vi "AVQ8347 Wavelike Data_backslash_n.vi"(0 "VISA Session":refnum<visa-resource-name>, 1 "Axis Select":T1(ring), 5 "Error In":errorcluster) -> (14 "Copy VISA Session":refnum<visa-resource-name>, 15 "Return All Data":string, 16 "Wavelike Data":dbl[](array[numeric]) format="%.12f", 17 "Return Data Bytes":u16, 19 "Error Out":errorcluster)   [LabVIEW 2020]
doc: "This function returns the wavelike data value\n\n(NEC-PC Mode Data is Return All Data Only)"
panel:
  out "CntWk":u16
  out "String Work":string
  # "Wavelike Data"
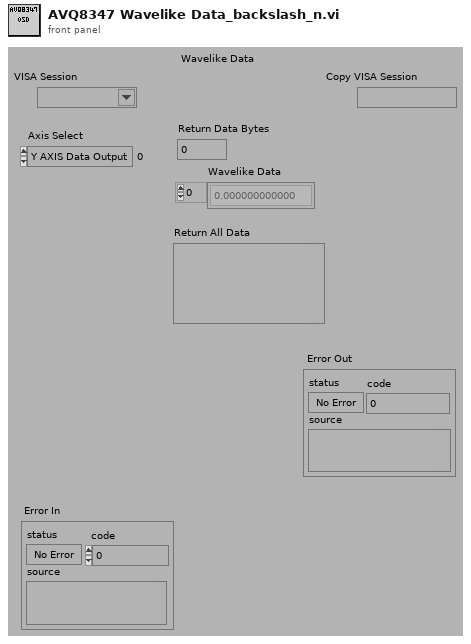
[diagram p1: front panel]
types:
  T1 = enum16{"Y AXIS Data Output", "X AXIS Data Output"}
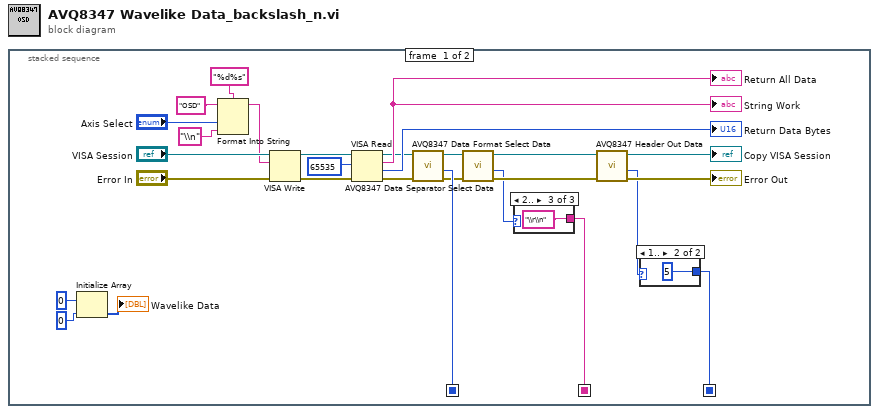
[diagram p0: block diagram]
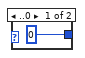
[diagram p2: hidden frame]
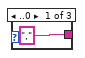
[diagram p3: hidden frame]
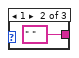
[diagram p4: hidden frame]
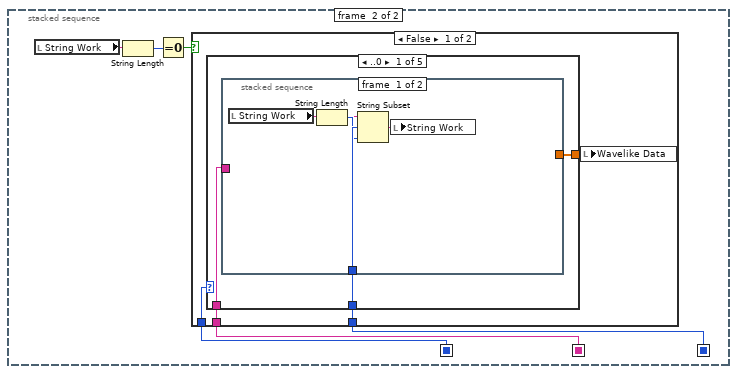
[diagram p5: hidden frame]
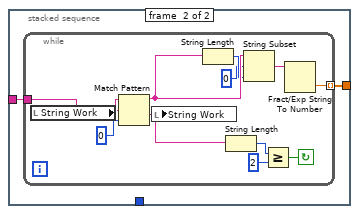
[diagram p6: hidden frame]
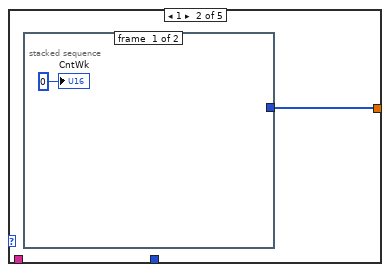
[diagram p7: hidden frame]
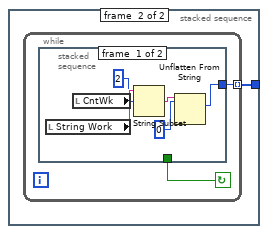
[diagram p8: hidden frame]
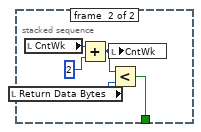
[diagram p9: hidden frame]
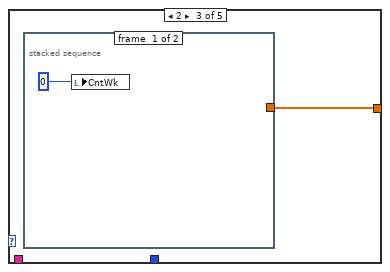
[diagram p10: hidden frame]
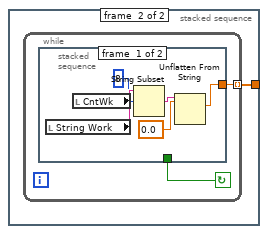
[diagram p11: hidden frame]
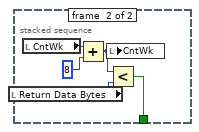
[diagram p12: hidden frame]
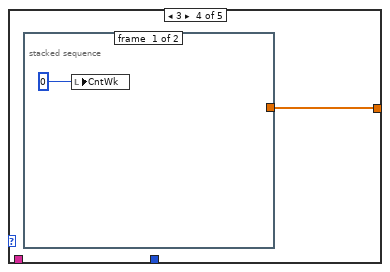
[diagram p13: hidden frame]
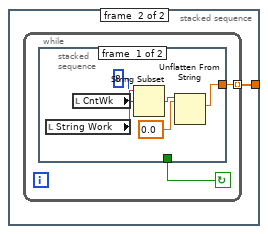
[diagram p14: hidden frame]
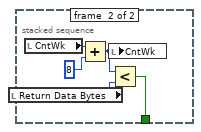
[diagram p15: hidden frame]
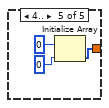
[diagram p16: hidden frame]
diagram:
  n1 = stacked-sequence {
    seq-local: [w18 _] -> [_ w36]
    seq-local: [w23 _] -> [_ w34]
    seq-local: [w12 _] -> [_ w35]
    frame #0 {
      n2 = Initialize Array(0, 0) -> (→"Wavelike Data":i32[])
      n3 = Format Into String(format string="%d%s", initial string="OSD", "Axis Select", "\\n") -> (resulting string=w14:string)  [unwired: 1 in, 1 out]
      n4 = VISA Write(VISA resource name="VISA Session", write buffer=w14, error in (no error)="Error In") -> (VISA resource name out=w24:refnum<visa-resource-name>, error out=w25:errorcluster)  [unwired: 1 out]
      n5 = VISA Read(VISA resource name=w24, byte count=65535, error in (no error)=w25) -> (VISA resource name out=w3:refnum<visa-resource-name>, read buffer=→"String Work" →"Return All Data":string, return count=→"Return Data Bytes":u32, error out=w2:errorcluster)
      n6 = call "AVQ8347 Data Format Select Data.vi"("Error In"=w2, "VISA Session"=w3) -> ("Error Out"=w11:errorcluster, "Data Format Select Value"=w12:u16, "Copy VISA Session"=w13:refnum<visa-resource-name>)  [unwired: 6 in, 1 out]
      n7 = call "AVQ8347 Data Separator Select Data.vi"("Error In"=w11, "VISA Session"=w13) -> ("Error Out"=w10:errorcluster, "Data Separrator Select Value"=w8:u16, "Copy VISA Session"=w9:refnum<visa-resource-name>)  [unwired: 6 in, 1 out]
      n8 = case shown="2.." w8 {
        tunnel: ["," " " "\\r\\n"] -> w18
        frame ..0 {
        }
        frame 1 {
        }
        frame 2.. {
        }
      }
      n9 = call "AVQ8347 Header Out Data.vi"("Error In"=w10, "VISA Session"=w9) -> ("Error Out"=→"Error Out":errorcluster, "Header Data Out Control Value"=w5:u16, "Copy VISA Session"=→"Copy VISA Session":refnum<visa-resource-name>)  [unwired: 6 in, 1 out]
      n10 = case shown="1.." w5 {
        tunnel: [0 5] -> w23
        frame ..0 {
        }
        frame 1.. {
        }
      }
    }
    frame #1 {
      n11 = local read "String Work"() -> (w39:string)
      n12 = String Length(string=w39) -> (length=w38:i32)
      n13 = Equal To 0?(x=w38) -> (x = 0?=w37:bool)
      n14 = case shown="False" w37 {
        tunnel: w36 -> [w43 _]
        tunnel: w35 -> [w42 _]
        tunnel: w34 -> [w41 _]
        frame False {
          n15 = case shown="..0" w42 {
            tunnel: w43 -> [w46 _ _ _ _]
            tunnel: w41 -> [w45 _ _ _ _]
            tunnel: [w44 w65 w81 w97 w113] -> w40
            frame ..0 {
              n16 = stacked-sequence {
                tunnel: w45 -> [w50 _]
                tunnel: w46 -> [_ w52]
                tunnel: [_ w51] -> w44
                frame #0 {
                  n17 = local read "String Work"() -> (w48:string)
                  n18 = String Length(string=w48) -> (length=w49:i32)
                  n19 = String Subset(string=w48, offset (0)=w50, length (rest)=w49) -> (substring=w47:string)
                  n20 = local write "String Work"(w47) -> ()
                }
                frame #1 {
                  n21 = while {
                    tunnel: [w59] -> w51 mode=indexing
                    tunnel: w52 -> [w58]
                    stop <- w55 continue-if-true
                    n22 = local read "String Work"() -> (w60:string)
                    n23 = Match Pattern(string=w60, regular expression=w58, offset (0)=0) -> (before substring=w63:string, after substring=w61:string)  [unwired: 2 out]
                    n24 = local write "String Work"(w61) -> ()
                    n25 = String Length(string=w63) -> (length=w62:i32)
                    n26 = String Length(string=w61) -> (length=w56:i32)
                    n27 = String Subset(string=w63, offset (0)=0, length (rest)=w62) -> (substring=w64:string)
                    n28 = Greater Or Equal?(x=w56, y=2) -> (x >= y?=w55:bool)
                    n29 = Fract/Exp String To Number(string=w64) -> (number=w59:dbl)  [unwired: 3 in, 1 out]
                  }
                }
              }
            }
            frame 1 {
              n30 = stacked-sequence {
                tunnel: [_ w67] -> w65
                frame #0 {
                  "CntWk" <- 0
                }
                frame #1 {
                  n31 = while {
                    tunnel: [w68] -> w67 mode=indexing
                    stop <- w69 continue-if-true
                    n32 = stacked-sequence {
                      tunnel: [_ w78] -> w69
                      tunnel: [w72 _] -> w68
                      frame #0 {
                        n33 = local read "String Work"() -> (w75:string)
                        n34 = local read "CntWk"() -> (w74:u16)
                        n35 = String Subset(string=w75, offset (0)=w74, length (rest)=2) -> (substring=w73:string)
                        n36 = Unflatten From String(type=u16 0, binary string=w73) -> (value=w72:u16)  [unwired: 3 in, 2 out]
                      }
                      frame #1 {
                        n37 = local read "Return Data Bytes"() -> (w76:u16)
                        n38 = local read "CntWk"() -> (w80:u16)
                        n39 = Add(x=w80, y=2) -> (x+y=w77:i32)
                        n40 = local write "CntWk"(w77) -> ()
                        n41 = Less?(x=w77, y=w76) -> (x < y?=w78:bool)
                      }
                    }
                  }
                }
              }
            }
            frame 2 {
              n42 = stacked-sequence {
                tunnel: [_ w83] -> w81
                frame #0 {
                  n43 = local write "CntWk"(0) -> ()
                }
                frame #1 {
                  n44 = while {
                    tunnel: [w84] -> w83 mode=indexing
                    stop <- w85 continue-if-true
                    n45 = stacked-sequence {
                      tunnel: [_ w94] -> w85
                      tunnel: [w88 _] -> w84
                      frame #0 {
                        n46 = local read "String Work"() -> (w91:string)
                        n47 = local read "CntWk"() -> (w90:u16)
                        n48 = String Subset(string=w91, offset (0)=w90, length (rest)=8) -> (substring=w89:string)
                        n49 = Unflatten From String(type=0.0, binary string=w89) -> (value=w88:dbl)  [unwired: 3 in, 2 out]
                      }
                      frame #1 {
                        n50 = local read "Return Data Bytes"() -> (w92:u16)
                        n51 = local read "CntWk"() -> (w96:u16)
                        n52 = Add(x=w96, y=8) -> (x+y=w93:i32)
                        n53 = local write "CntWk"(w93) -> ()
                        n54 = Less?(x=w93, y=w92) -> (x < y?=w94:bool)
                      }
                    }
                  }
                }
              }
            }
            frame 3 {
              n55 = stacked-sequence {
                tunnel: [_ w99] -> w97
                frame #0 {
                  n56 = local write "CntWk"(0) -> ()
                }
                frame #1 {
                  n57 = while {
                    tunnel: [w100] -> w99 mode=indexing
                    stop <- w101 continue-if-true
                    n58 = stacked-sequence {
                      tunnel: [_ w110] -> w101
                      tunnel: [w104 _] -> w100
                      frame #0 {
                        n59 = local read "String Work"() -> (w107:string)
                        n60 = local read "CntWk"() -> (w106:u16)
                        n61 = String Subset(string=w107, offset (0)=w106, length (rest)=8) -> (substring=w105:string)
                        n62 = Unflatten From String(type=sgl 0.0, binary string=w105) -> (value=w104:sgl)  [unwired: 3 in, 2 out]
                      }
                      frame #1 {
                        n63 = local read "Return Data Bytes"() -> (w108:u16)
                        n64 = local read "CntWk"() -> (w112:u16)
                        n65 = Add(x=w112, y=8) -> (x+y=w109:i32)
                        n66 = local write "CntWk"(w109) -> ()
                        n67 = Less?(x=w109, y=w108) -> (x < y?=w110:bool)
                      }
                    }
                  }
                }
              }
            }
            frame 4.. {
              n68 = Initialize Array(0, 0) -> (w113:i32[])
            }
          }
          n69 = local write "Wavelike Data"(w40) -> ()
        }
        frame True {
        }
      }
    }
  }
